vi "R1_DO Control.vi"(0 "Air Short Reaction Time (s)":dbl=0.05, 1 "N2 Gain":dbl=0.01, 3 "DO Tolerance (mg/L)":dbl=0.05, 4 "Long Reaction Time (s)":dbl=0.05, 5 "Air Gain":dbl=0.01, 6 "N2 Short Reaction Time (s)":dbl=0.05, 7 "DO Set Point (mg/L)":dbl=0.05) -> ()   [LabVIEW 2016]
uses:
  R2 DO Manual Control.ctl
  R2 Reactor Status v1.ctl
  R2Variables.lvlib
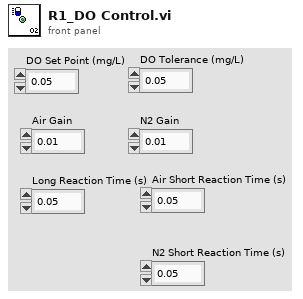
[diagram p1: front panel]
types:
  T1 = typedef "R2Variables.lvlib/R2 DO Manual Control.ctl" = cluster{"Air Valve":bool, "N2 Valve":bool}
  T2 = typedef "R2Variables.lvlib/R2 Reactor Status v1.ctl" = cluster{"Water Pump":bool, "Media Pump":bool, "Effluent Pump":bool, "Base Pump":bool, "Gas Pump":bool, "Acid Pump":bool, "Air Release Valve":bool, "N2 Valve":bool, "pH":dbl, "DO (mg/L)":dbl, "pH Amp (A)":dbl, "DO Amp (A)":dbl, "Release Flow":dbl, "Compressed Air":dbl, "Reactor Status":sgl, "Air Valve":bool}
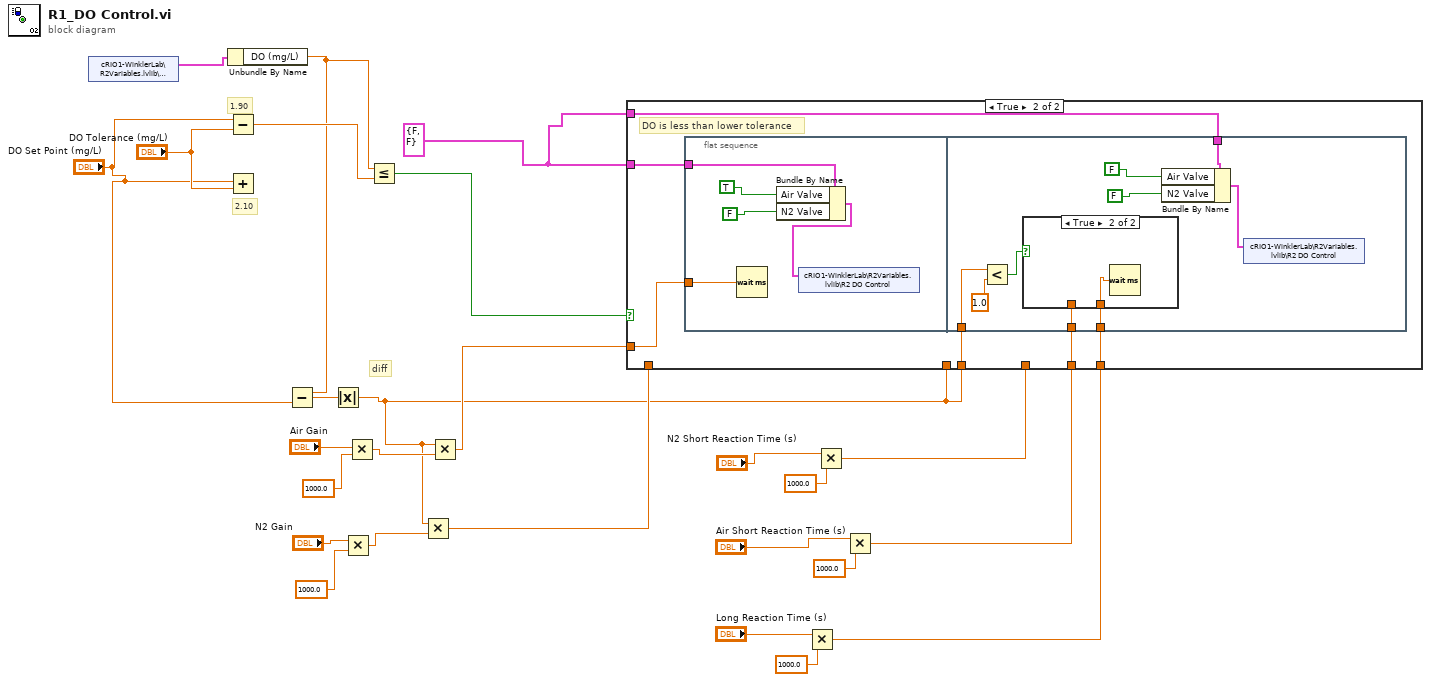
[diagram p0: block diagram]
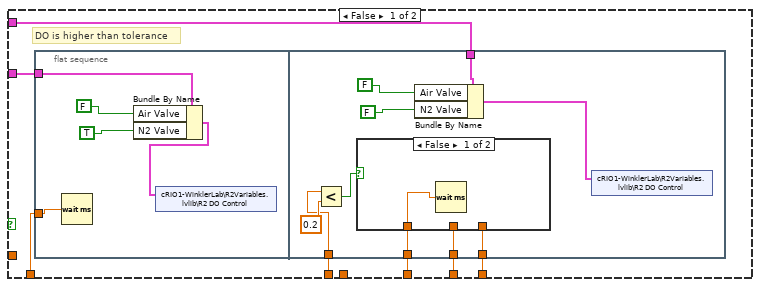
[diagram p2: hidden frame]
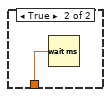
[diagram p3: hidden frame]
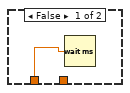
[diagram p4: hidden frame]
diagram:
  w7 = T1 {"Air Valve"=FALSE, "N2 Valve"=FALSE} ("Reactor 2 DO Control")
  # "2.10"
  # "1.90"
  # "diff"
  n1 = shared-variable "cRIO1-WinklerLab\\R2Variables.lvlib\\R2Status"() -> (w26:T2)  [unwired: 1 in, 1 out]
  n2 = Unbundle By Name(w26) -> ("DO (mg/L)"=w19:dbl)
  n3 = Subtract(x="DO Set Point (mg/L)", y="DO Tolerance (mg/L)") -> (x-y=w20:dbl)
  n4 = Add(x="DO Set Point (mg/L)", y="DO Tolerance (mg/L)") -> ()  [unwired: 1 out]
  n5 = Subtract(x=w19, y="DO Set Point (mg/L)") -> (x-y=w24:dbl)
  n6 = Absolute Value(x=w24) -> (abs(x)=w3:dbl)
  n7 = Multiply(x="N2 Gain", y=1000.0) -> (x*y=w17:dbl)
  n8 = Multiply(x="Air Gain", y=1000.0) -> (x*y=w16:dbl)
  n9 = Less Or Equal?(x=w19, y=w20) -> (x <= y?=w18:bool)
  n10 = Multiply(x=w3, y=w17) -> (x*y=w8:dbl)
  n11 = Multiply(x=w3, y=w16) -> (x*y=w15:dbl)
  n12 = Multiply(x="Long Reaction Time (s)", y=1000.0) -> (x*y=w1:dbl)
  n13 = Multiply(x="N2 Short Reaction Time (s)", y=1000.0) -> (x*y=w2:dbl)
  n14 = Multiply(x="Air Short Reaction Time (s)", y=1000.0) -> (x*y=w4:dbl)
  n15 = case shown="True" w18 {
    tunnel: w7 -> [w33 w55]
    tunnel: w15 -> [_ w56]
    tunnel: w8 -> [w32 _]
    tunnel: w7 -> [w31 w54]
    tunnel: w3 -> [w30 _]
    tunnel: w4 -> [w28 w53]
    tunnel: w3 -> [_ w52]
    tunnel: w2 -> [w29 _]
    tunnel: w1 -> [w27 w51]
    frame False {
      # "DO is higher than tolerance"
      n16 = flat-sequence {
        tunnel: w33 -> [w38]
        tunnel: w32 -> [w37]
        tunnel: w31 -> [w46]
        tunnel: w30 -> [w42]
        tunnel: w29 -> [w41]
        tunnel: w28 -> [w40]
        tunnel: w27 -> [w39]
        frame #0 {
          n17 = Wait (ms)(milliseconds to wait=w37) -> ()  [unwired: 1 out]
          n18 = Bundle By Name(cluster=w38, "Air Valve"=FALSE, "N2 Valve"=TRUE) -> (w34:T1)
          n19 = shared-variable "cRIO1-WinklerLab\\R2Variables.lvlib\\R2 DO Control"(w34) -> ()  [unwired: 1 in, 1 out]
        }
        frame #1 {
          n20 = Less?(x=w42, y=0.2) -> (x < y?=w43:bool)
          n21 = case shown="False" w43 {
            tunnel: w41 -> [w49 _]
            tunnel: w40 -> [_ _]
            tunnel: w39 -> [_ w50]
            frame False {
              n22 = Wait (ms)(milliseconds to wait=w49) -> ()  [unwired: 1 out]
            }
            frame True {
              n23 = Wait (ms)(milliseconds to wait=w50) -> ()  [unwired: 1 out]
            }
          }
          n24 = Bundle By Name(cluster=w46, "Air Valve"=FALSE, "N2 Valve"=FALSE) -> (w45:T1)
          n25 = shared-variable "cRIO1-WinklerLab\\R2Variables.lvlib\\R2 DO Control"(w45) -> ()  [unwired: 1 in, 1 out]
        }
      }
    }
    frame True {
      # "DO is less than lower tolerance"
      n26 = flat-sequence {
        tunnel: w56 -> [w61]
        tunnel: w55 -> [w60]
        tunnel: w54 -> [w65]
        tunnel: w53 -> [w64]
        tunnel: w52 -> [w63]
        tunnel: w51 -> [w62]
        frame #0 {
          n27 = Wait (ms)(milliseconds to wait=w61) -> ()  [unwired: 1 out]
          n28 = Bundle By Name(cluster=w60, "Air Valve"=TRUE, "N2 Valve"=FALSE) -> (w57:T1)
          n29 = shared-variable "cRIO1-WinklerLab\\R2Variables.lvlib\\R2 DO Control"(w57) -> ()  [unwired: 1 in, 1 out]
        }
        frame #1 {
          n30 = Less?(x=w63, y=1.0) -> (x < y?=w70:bool)
          n31 = case shown="True" w70 {
            tunnel: w64 -> [w71 _]
            tunnel: w62 -> [_ w72]
            frame False {
              n32 = Wait (ms)(milliseconds to wait=w71) -> ()  [unwired: 1 out]
            }
            frame True {
              n33 = Wait (ms)(milliseconds to wait=w72) -> ()  [unwired: 1 out]
            }
          }
          n34 = Bundle By Name(cluster=w65, "Air Valve"=FALSE, "N2 Valve"=FALSE) -> (w66:T1)
          n35 = shared-variable "cRIO1-WinklerLab\\R2Variables.lvlib\\R2 DO Control"(w66) -> ()  [unwired: 1 in, 1 out]
        }
      }
    }
  }
